vi "Extract first matched pixels.vi"(9 "Side":enum16{"Top", "Left", "Bottom", "Right"}(ring), 10 "Dimensions":cluster{i32, i32}={640, 480}, 11 "Image Pixels (U8)":u8[][](array[numeric])) -> (2 "Y out":i16[](array[numeric]), 3 "X out":i16[](array[numeric]))   [LabVIEW 2012]
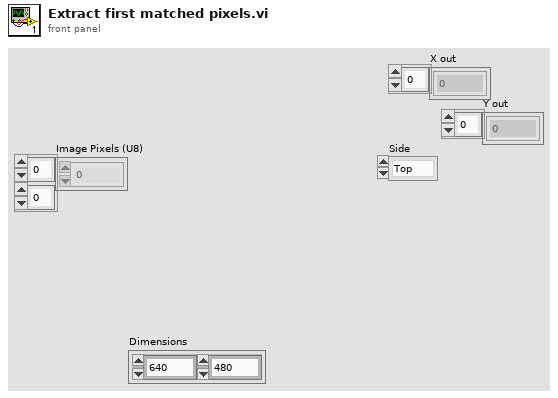
[diagram p1: front panel]
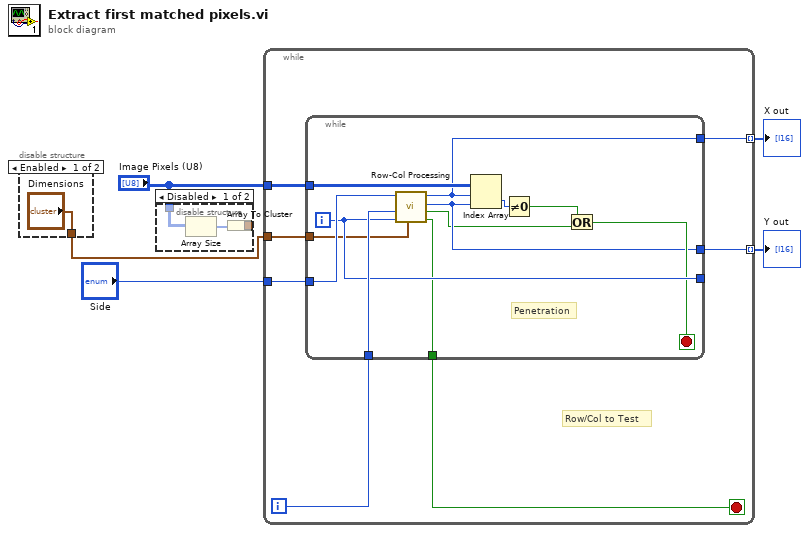
[diagram p0: block diagram]
diagram:
  n1 = disable-structure shown="Enabled" {
    disable-tunnel: ["Dimensions" _] -> w1
    frame Enabled {
    }
    frame Disabled {
    }
  }
  n2 = disable-structure shown="Disabled" {
    disable-tunnel: "Image Pixels (U8)" -> [w8 _]
    disable-tunnel: [w7 _] -> _
    frame Disabled {
      n3 = Array Size(array=w8) -> (size(s)=w9:i32[])
      n4 = Array To Cluster(array=w9) -> (cluster=w7:cluster{"[0]":i32, "[1]":i32})
    }
    frame Enabled {
    }
  }
  n5 = while {
    tunnel: "Image Pixels (U8)" -> [w15]
    tunnel: "Side" -> [w14]
    tunnel: [w13] -> w4 mode=indexing
    tunnel: [w12] -> w3 mode=indexing
    tunnel: w1 -> [w10]
    i -> [w16]
    stop <- w11 stop-if-true
    # "Row/Col to Test"
    n6 = while {
      tunnel: w16 -> [w27]
      tunnel: w15 -> [w24]
      tunnel: [w26] -> _
      tunnel: w14 -> [w28]
      tunnel: [w21] -> w13
      tunnel: [w20] -> w12
      tunnel: [w18] -> w11
      tunnel: w10 -> [w17]
      i -> [w26]
      stop <- w25 stop-if-true
      # "Penetration"
      n7 = call "Row-Col Processing.vi"("Array bounds"=w17, "Penetration"=w26, "Row/Col to test"=w27, "Side"=w28) -> ("Last Row/Column?"=w18:bool, "Done?"=w19:bool, "X"=w20:i16, "Y"=w21:i16)  [unwired: 3 in]
      n8 = Index Array(array=w24, index (row)=w21, index (col)=w20) -> (element=w23:u8)
      n9 = Not Equal To 0?(x=w23) -> (x != 0?=w22:bool)
      n10 = Or(x=w22, y=w19) -> (x .or. y?=w25:bool)
    }
  }
  "X out" <- w4
  "Y out" <- w3
